vi "Configure Active Trace.vi"(5 "Format":T1, 7 "S parameter":T2(ring), 8 "error in (no error)":errorcluster, 10 "Active Trace":u8=1, 11 "VNA-PNA in":refnum<class "VNA-PNA.lvclass">) -> (0 "error out":errorcluster, 3 "VNA-PNA out":refnum<class "VNA-PNA.lvclass">)   [LabVIEW 2020, in "VNA-PNA.lvclass"]
doc: "Configures the active trace.\nIt creates the trace and sets the S paramert and mode."
uses:
  VNA-PNA.lvclass
  C:/Sandbox/RF Bench/Source Code/WiSpry Test Framework/Instruments/Vector Network Analyzer/Vector Network Analyzer.lvclass
  C:/Sandbox/RF Bench/Source Code/WiSpry Test Framework/Instruments/Instrument.lvclass
  Controls/S parm format enum.ctl
  Vector Network Analyzer.lvclass/Vector Network Analyzer.ctl
  Instrument.lvclass/Instrument.ctl
  Vector Network Analyzer.lvclass
  Instrument.lvclass
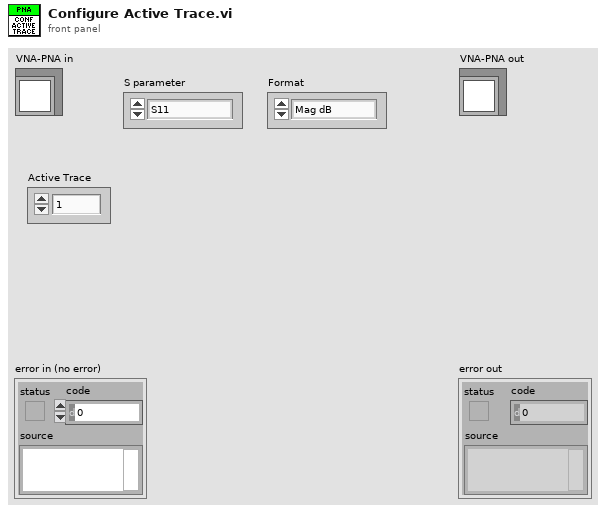
[diagram p1: front panel]
types:
  T1 = typedef "Vector Network Analyzer.lvclass/S parm format enum.ctl" = enum16{"Mag dB", "Mag", "Phase", "Smith", "Real", "Imag", "Group Delay", "SWR"}
  T2 = enum16{"S11", "S21", "S31", "S41", "S22", "S12", "S32", "S42", "S33", "S13", "S23", "S43", "S44", "S14", "S24", "S34"}
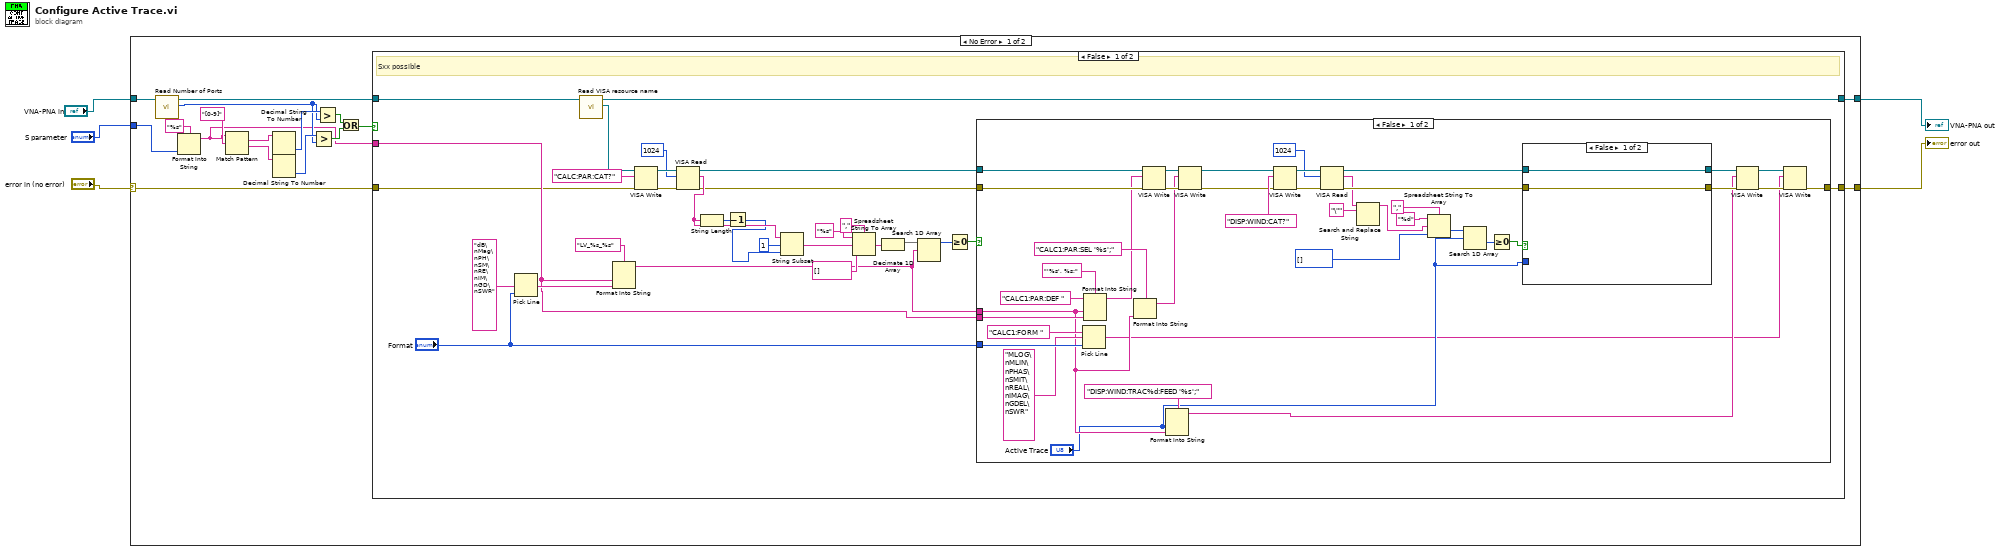
[diagram p0: block diagram]
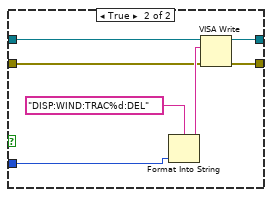
[diagram p2: hidden frame]
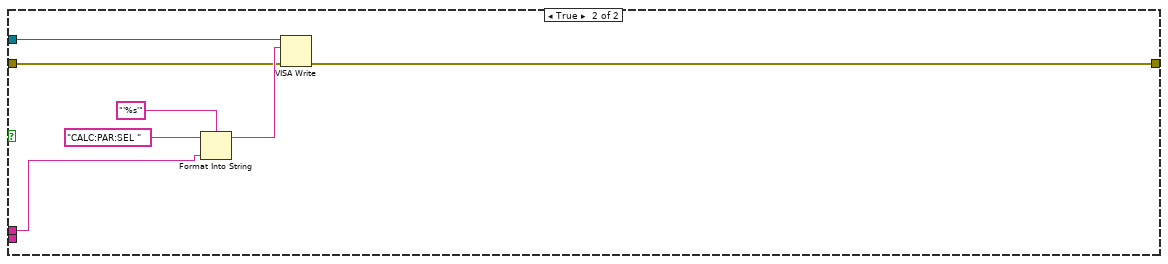
[diagram p3: hidden frame]
diagram:
  n1 = case shown="No Error" "error in (no error)" {
    selector: "error in (no error)" -> [w9 w111]
    tunnel: "VNA-PNA in" -> [w22 w110]
    tunnel: "S parameter" -> [w20 _]
    tunnel: [w7 w111] -> w2
    tunnel: [w6 w110] -> w1
    frame No Error {
      n2 = call "Read Number of Ports.vi"("Vector Network Analyzer in"=w22) -> ("Number of Ports"=w14:i32, "Vector Network Analyzer out"=w10:refnum<class "VNA-PNA.lvclass">)  [unwired: 9 in]
      n3 = Format Into String(format string="%s", w20) -> (resulting string=w8:string)  [unwired: 2 in, 1 out]
      n4 = Match Pattern(string=w8, regular expression="[0-9]") -> (match substring=w18:string, after substring=w17:string)  [unwired: 1 in, 2 out]
      n5 = Decimal String To Number(string=w18) -> (number=w16:i32)  [unwired: 2 in, 1 out]
      n6 = Decimal String To Number(string=w17) -> (number=w15:i32)  [unwired: 2 in, 1 out]
      n7 = Greater?(x=w15, y=w14) -> (0:w12:bool)
      n8 = Greater?(x=w16, y=w14) -> (0:w13:bool)
      n9 = Or(x=w13, y=w12) -> (x .or. y?=w11:bool)
      n10 = case shown="False" w11 {
        tunnel: w10 -> [w50 w109]
        tunnel: w9 -> [w42 w108]
        tunnel: w8 -> [w45 _]
        tunnel: [w46 w108] -> w7
        tunnel: [w49 w109] -> w6
        frame False {
          # "Sxx possible"
          n11 = Pick Line(multi-line string="dB\nMag\nPH\nSM\nRE\nIM\nGD\nSWR", line index="Format") -> (output string=w47:string)  [unwired: 1 in]
          n12 = call "Read VISA resource name.vi"("Instrument in"=w50) -> ("VISA resource name"=w43:refnum<visa-resource-name>, "Instrument out"=w49:refnum<class "VNA-PNA.lvclass">)  [unwired: 9 in]
          n13 = Format Into String(format string="LV_%s_%s" ("initial string"), w45, w47) -> (resulting string=w24:string)  [unwired: 2 in, 1 out]
          n14 = VISA Write(VISA resource name=w43, write buffer="CALC:PAR:CAT?", error in (no error)=w42) -> (VISA resource name out=w39:refnum<visa-resource-name>, error out=w40:errorcluster)  [unwired: 1 out]
          n15 = VISA Read(VISA resource name=w39, byte count=u32 1024, error in (no error)=w40) -> (VISA resource name out=w25:refnum<visa-resource-name>, read buffer=w34:string, error out=w27:errorcluster)  [unwired: 1 out]
          n16 = String Length(string=w34) -> (length=w35:i32)
          n17 = Decrement(x=w35) -> (x-1=w32:i32)
          n18 = String Subset(string=w34, offset (0)=1, length (rest)=w32) -> (substring=w31:string)
          n19 = Spreadsheet String To Array(delimiter (Tab)=",", format string="%s", spreadsheet string=w31, array type (2D Dbl)=string[] []) -> (array=w28:string[])
          n20 = Decimate 1D Array(w28) -> (w23:string[])  [unwired: 1 out]
          n21 = Search 1D Array(1D array=w23, element=w24) -> (index of element=w29:i32)  [unwired: 1 in]
          n22 = Greater Or Equal To 0?(x=w29) -> (x >= 0?=w26:bool)
          n23 = case shown="False" w26 {
            tunnel: [w55 w101] -> w46
            tunnel: w45 -> [w91 _]
            tunnel: "Format" -> [w90 _]
            tunnel: w24 -> [w83 w104]
            tunnel: w27 -> [w82 w103]
            tunnel: w25 -> [w81 w102]
            frame False {
              n24 = Pick Line(string ("")="CALC1:FORM ", multi-line string="MLOG\nMLIN\nPHAS\nSMIT\nREAL\nIMAG\nGDEL\nSWR", line index=w90) -> (output string=w52:string)
              n25 = Format Into String(format string="'%s', %s;", initial string="CALC1:PAR:DEF ", w83, w91) -> (resulting string=w80:string)  [unwired: 1 in, 1 out]
              n26 = Format Into String(format string="CALC1:PAR:SEL '%s';", w83) -> (resulting string=w77:string)  [unwired: 2 in, 1 out]
              n27 = VISA Write(VISA resource name=w81, write buffer=w80, error in (no error)=w82) -> (VISA resource name out=w78:refnum<visa-resource-name>, error out=w79:errorcluster)  [unwired: 1 out]
              n28 = Format Into String(format string="DISP:WIND:TRAC%d:FEED '%s';" ("write buffer"), "Active Trace", w83) -> (resulting string=w56:string)  [unwired: 2 in, 1 out]
              n29 = VISA Write(VISA resource name=w78, write buffer=w77, error in (no error)=w79) -> (VISA resource name out=w57:refnum<visa-resource-name>, error out=w58:errorcluster)  [unwired: 1 out]
              n30 = VISA Write(VISA resource name=w57, write buffer="DISP:WIND:CAT?", error in (no error)=w58) -> (VISA resource name out=w74:refnum<visa-resource-name>, error out=w75:errorcluster)  [unwired: 1 out]
              n31 = VISA Read(VISA resource name=w74, byte count=u32 1024, error in (no error)=w75) -> (VISA resource name out=w67:refnum<visa-resource-name>, read buffer=w61:string, error out=w66:errorcluster)  [unwired: 1 out]
              n32 = Search and Replace String(input string=w61, search string="\"") -> (result string=w60:string)  [unwired: 6 in, 3 out]
              n33 = Spreadsheet String To Array(delimiter (Tab)=",", format string="%d", spreadsheet string=w60, array type (2D Dbl)=i32[] []) -> (array=w70:i32[])
              n34 = Search 1D Array(1D array=w70, element="Active Trace") -> (index of element=w69:i32)  [unwired: 1 in]
              n35 = Greater Or Equal To 0?(x=w69) -> (x >= 0?=w68:bool)
              n36 = case shown="False" w68 {
                tunnel: w67 -> [w92 w95]
                tunnel: w66 -> [w93 w96]
                tunnel: [w93 w98] -> w65
                tunnel: [w92 w94] -> w64
                tunnel: "Active Trace" -> [_ w99]
                frame False {
                }
                frame True {
                  n37 = Format Into String(format string="DISP:WIND:TRAC%d:DEL", w99) -> (resulting string=w97:string)  [unwired: 2 in, 1 out]
                  n38 = VISA Write(VISA resource name=w95, write buffer=w97, error in (no error)=w96) -> (VISA resource name out=w94:refnum<visa-resource-name>, error out=w98:errorcluster)  [unwired: 1 out]
                }
              }
              n39 = VISA Write(VISA resource name=w64, write buffer=w56, error in (no error)=w65) -> (VISA resource name out=w53:refnum<visa-resource-name>, error out=w54:errorcluster)  [unwired: 1 out]
              n40 = VISA Write(VISA resource name=w53, write buffer=w52, error in (no error)=w54) -> (error out=w55:errorcluster)  [unwired: 2 out]
            }
            frame True {
              n41 = Format Into String(format string="'%s'", initial string="CALC:PAR:SEL ", w104) -> (resulting string=w105:string)  [unwired: 1 in, 1 out]
              n42 = VISA Write(VISA resource name=w102, write buffer=w105, error in (no error)=w103) -> (error out=w101:errorcluster)  [unwired: 2 out]
            }
          }
        }
        frame True {
          # "Add error handler"
          # "Sxx higher than ports"
        }
      }
    }
    frame Error {
    }
  }
  "error out" <- w2
  "VNA-PNA out" <- w1
